vi "运维调试.vi"() -> ()   [LabVIEW 2016]
uses:
  <vilib>/Utility/miscctls.llb/LVPointTypeDef.ctl
  PLC/PLC.lvlib
  <vilib>/Utility/config.llb/NI_LVConfig.lvlib
panel:
  in  "运维调试菜单":T1(xcontrol)
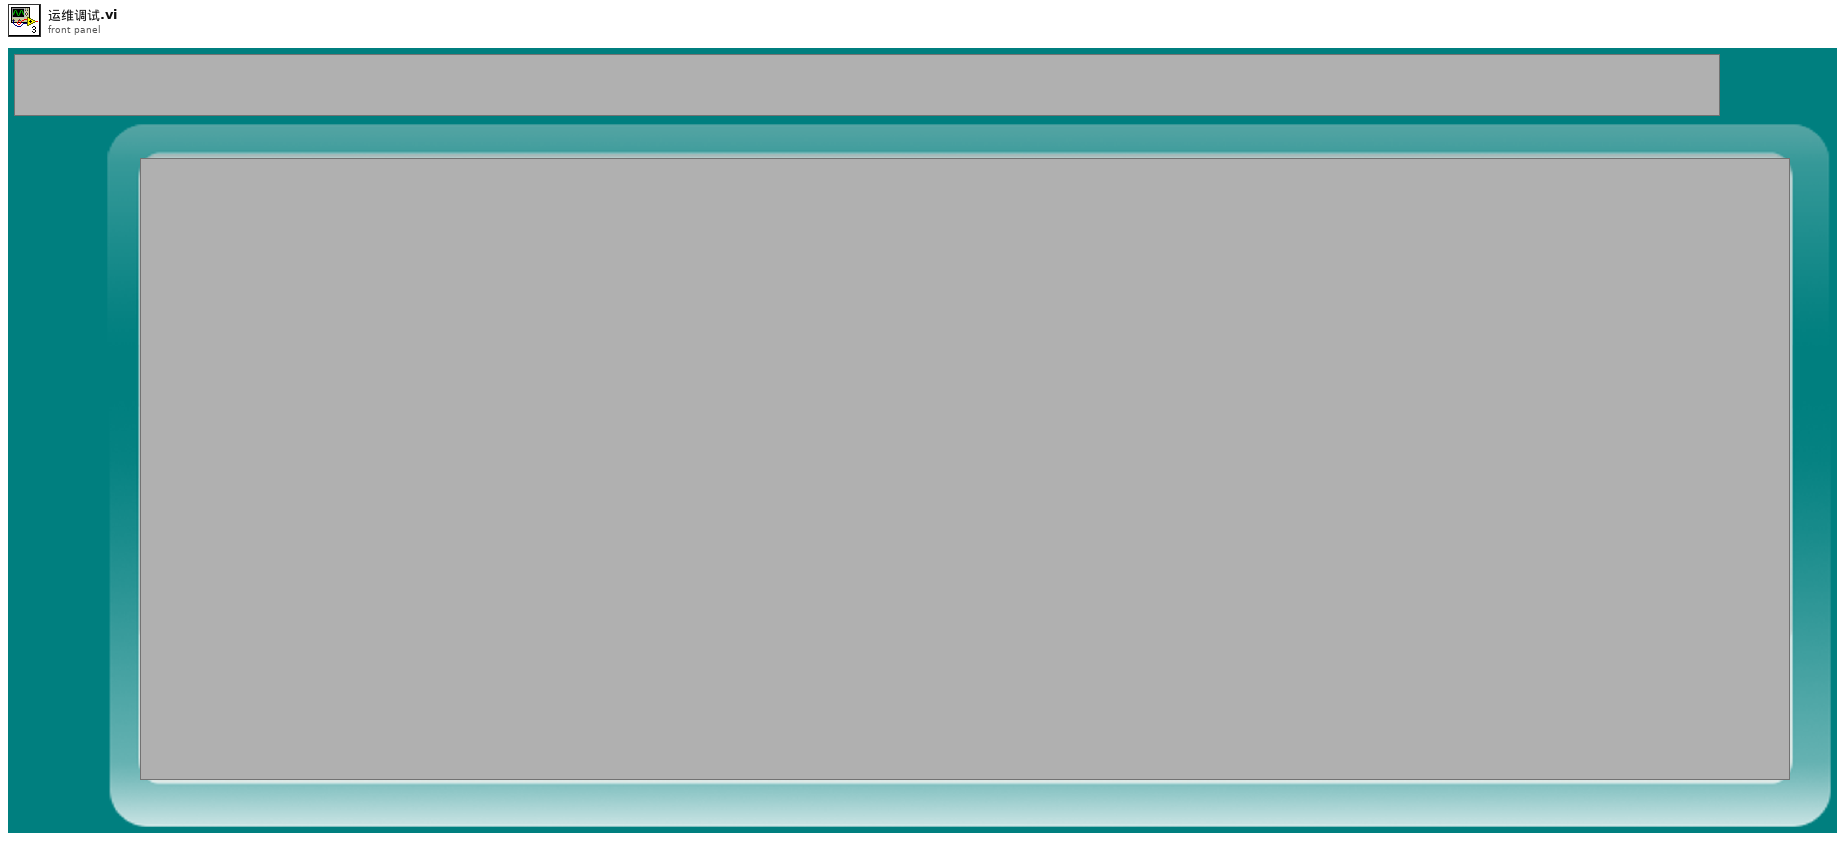
[diagram p1: front panel]
types:
  T1 = enum16{"电源管理", "采配水", "氨氮", "总磷总氮", "多参数", "CODMn", "CODcr", "流量计", "质控单元", "其他"}
  T2 = typedef "NI_LVConfig.lvlib/Config Data RefNum.ctl" = refnum<k1>
  T3 = typedef "LVPointTypeDef.ctl" = cluster{"Horizontal":i16, "Vertical":i16}
  T4 = enum16{"Enabled", "Disabled", "Disabled and Grayed Out"}
  T5 = enum32{"Bad", "Idle", "Run top level", "Running"}
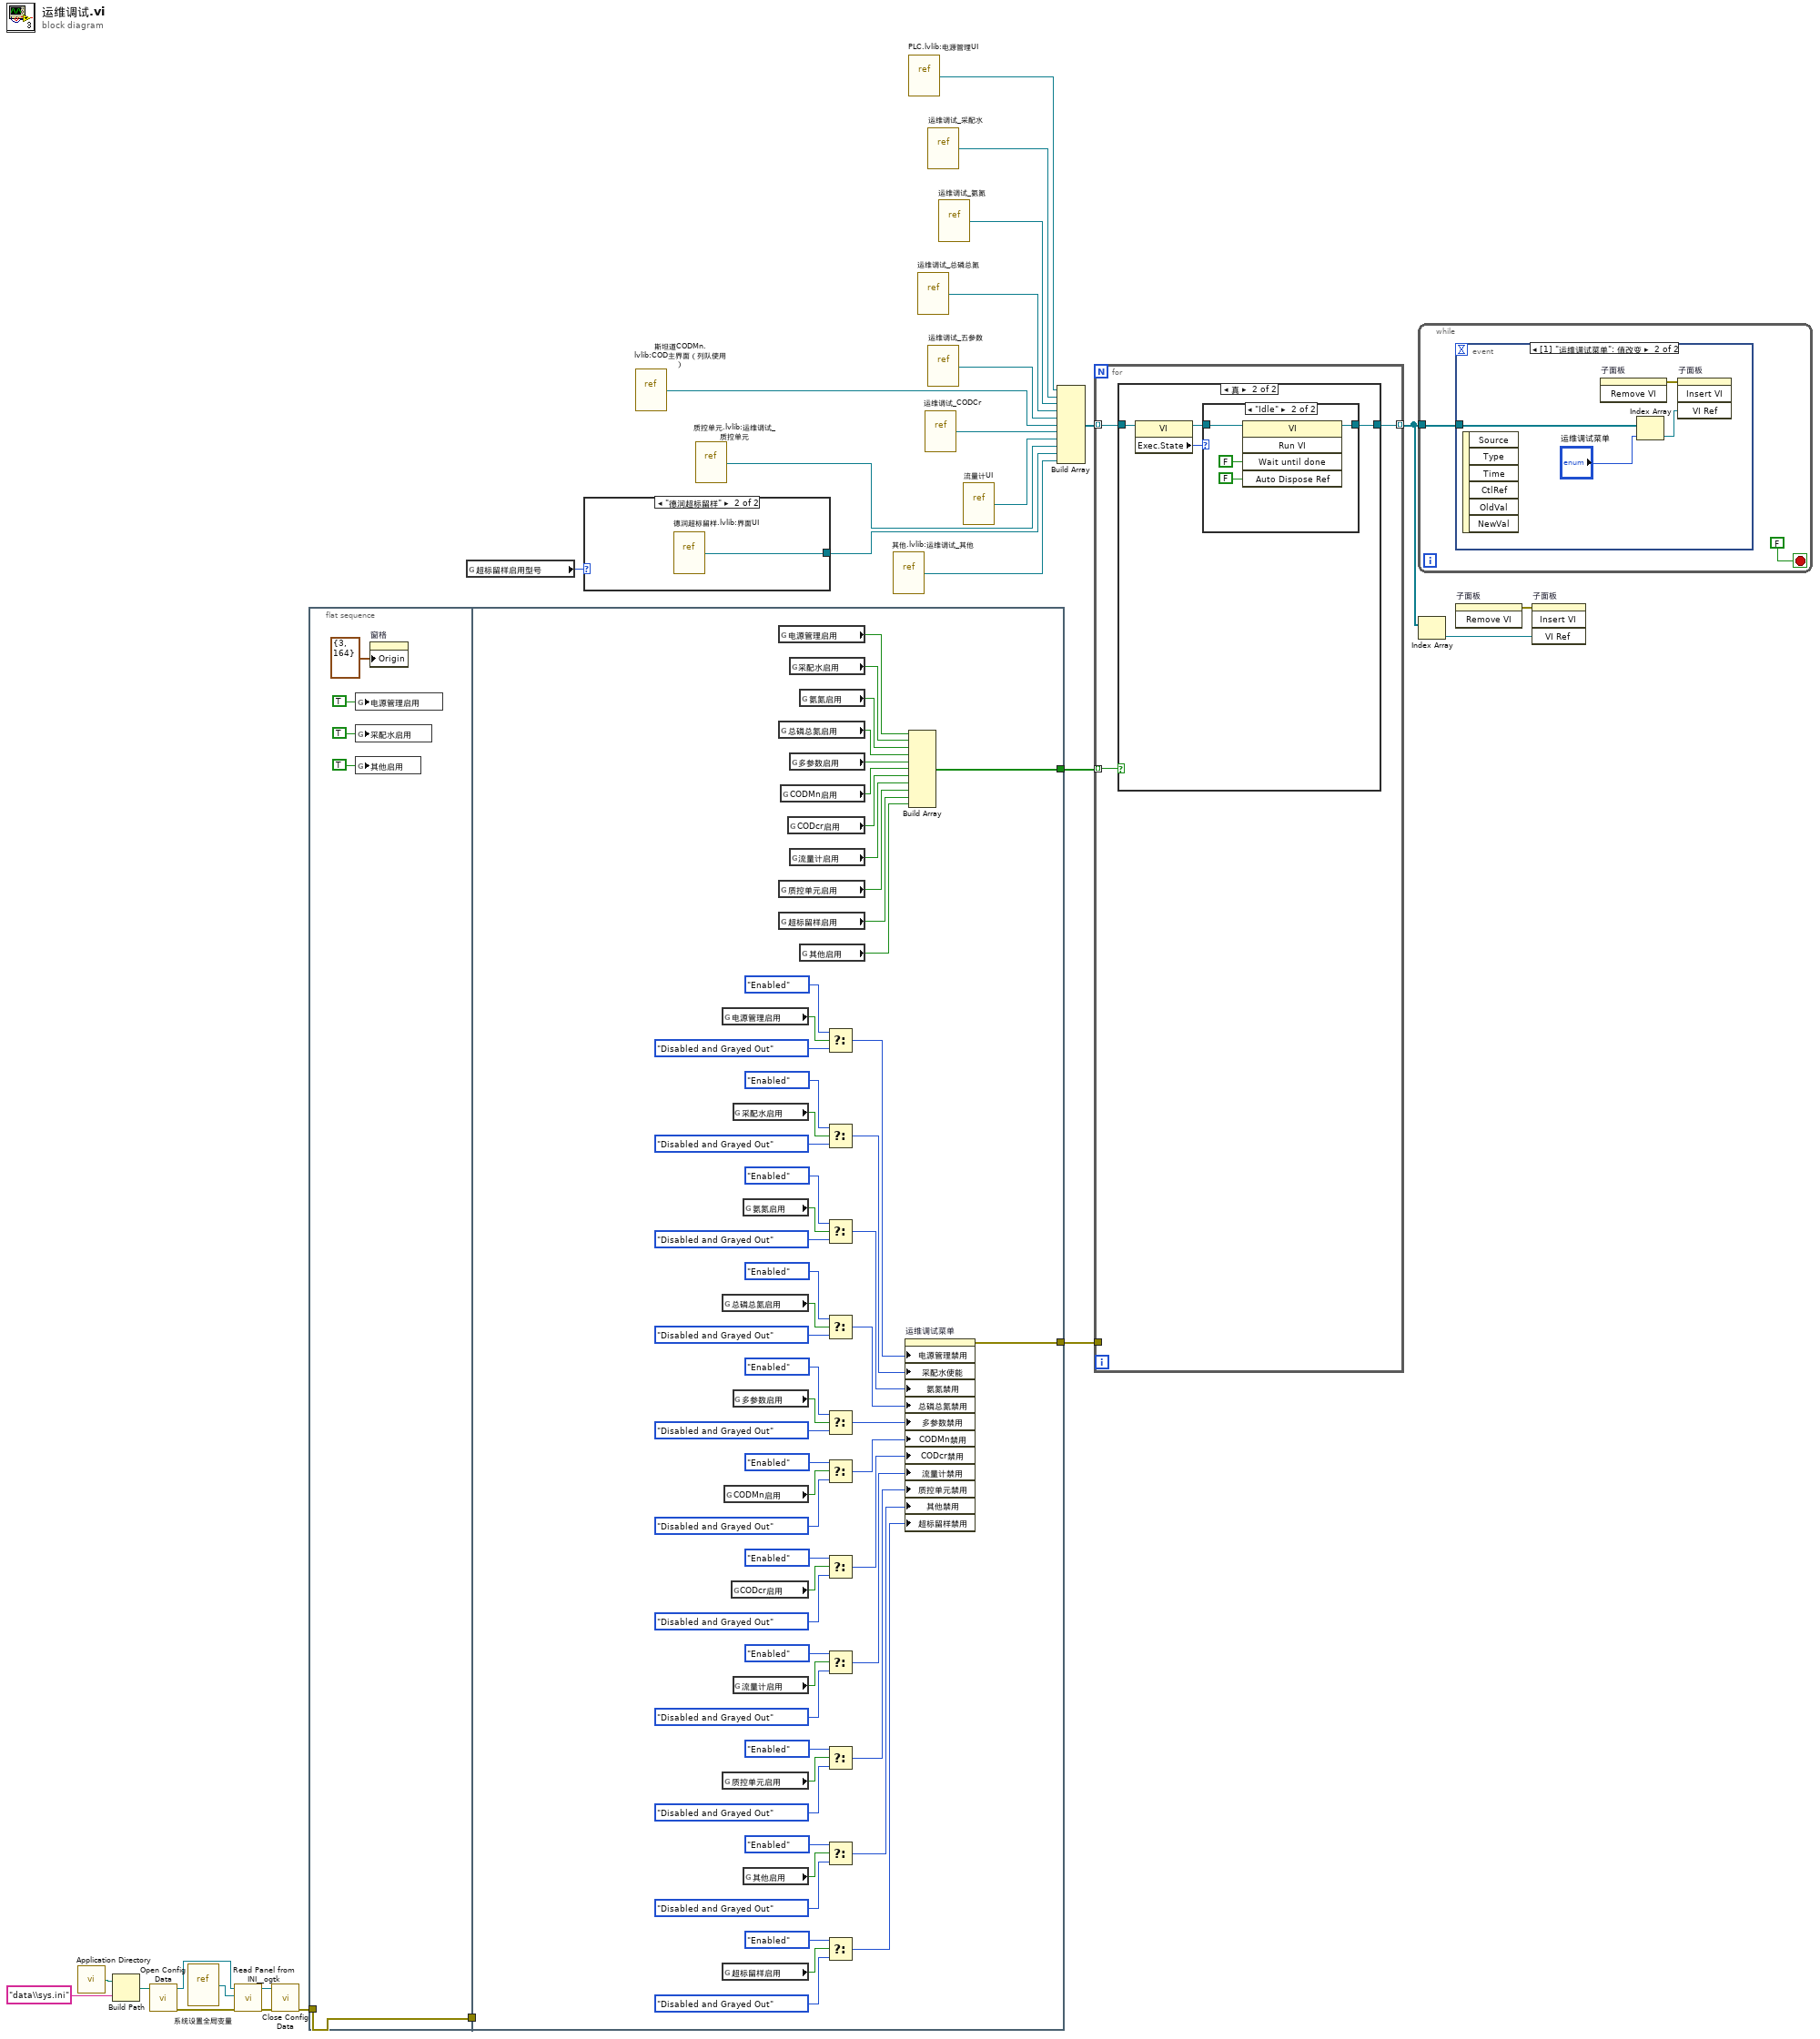
[diagram p0: block diagram]
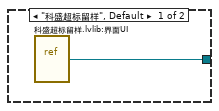
[diagram p2: hidden frame]
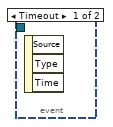
[diagram p5: hidden frame]
diagram:
  n1 = call <vilib>:"Application Directory.vi"() -> ("Application Directory"=w8:path)
  n2 = Build Path(base path=w8, name or relative path="data\\sys.ini" ("名称或相对路径")) -> (appended path=w6:path)
  n3 = call <vilib>:"Open Config Data.vi"("configuration file path"=w6) -> ("error out"=w15:errorcluster, "refnum"=w14:T2)  [unwired: 8 in, 1 out]
  n4 = vi-ref "系统设置全局变量.vi"() -> (w13:refnum<vi>)
  n5 = call <userlib>:"Read Panel from INI__ogtk.vi"("error in (no error)"=w15, "VI ref"=w13, "refnum"=w14) -> ("error out"=w12:errorcluster, "refnum out"=w11:T2)  [unwired: 7 in]
  n6 = call <vilib>:"Close Config Data.vi"("error in (no error)"=w12, "refnum"=w11) -> ("error out"=w10:errorcluster)  [unwired: 8 in, 1 out]
  n7 = flat-sequence {
    tunnel: w10 -> [w33]
    tunnel: [w33] -> w9
    tunnel: [w71] -> w16
    tunnel: w9 -> [_]
    tunnel: [w60] -> w5
    frame #0 {
      n8 = global write "系统设置全局变量.vi" "电源管理启用"(TRUE ("电源管理启用")) -> ()
      n9 = global write "系统设置全局变量.vi" "采配水启用"(TRUE ("采配水启用")) -> ()
      n10 = global write "系统设置全局变量.vi" "其他启用"(TRUE ("其他启用")) -> ()
      n11 = property on="窗格" class="Pane"("Origin"=T3 {"Horizontal"=3, "Vertical"=164} ("原点")) -> ()  [unwired: 2 in, 2 out]
    }
    frame #1 {
      n12 = global read "系统设置全局变量.vi" "电源管理启用"() -> (w90:bool)
      n13 = global read "系统设置全局变量.vi" "总磷总氮启用"() -> (w85:bool)
      n14 = global read "系统设置全局变量.vi" "质控单元启用"() -> (w78:bool)
      n15 = global read "系统设置全局变量.vi" "超标留样启用"() -> (w36:bool)
      n16 = global read "系统设置全局变量.vi" "CODMn启用"() -> (w81:bool)
      n17 = global read "系统设置全局变量.vi" "CODcr启用"() -> (w80:bool)
      n18 = global read "系统设置全局变量.vi" "采配水启用"() -> (w87:bool)
      n19 = global read "系统设置全局变量.vi" "多参数启用"() -> (w83:bool)
      n20 = global read "系统设置全局变量.vi" "流量计启用"() -> (w79:bool)
      n21 = global read "系统设置全局变量.vi" "氨氮启用"() -> (w39:bool)
      n22 = global read "系统设置全局变量.vi" "其他启用"() -> (w77:bool)
      n23 = global read "系统设置全局变量.vi" "电源管理启用"() -> (w61:bool)
      n24 = global read "系统设置全局变量.vi" "总磷总氮启用"() -> (w64:bool)
      n25 = global read "系统设置全局变量.vi" "质控单元启用"() -> (w69:bool)
      n26 = global read "系统设置全局变量.vi" "超标留样启用"() -> (w70:bool)
      n27 = global read "系统设置全局变量.vi" "CODMn启用"() -> (w66:bool)
      n28 = global read "系统设置全局变量.vi" "CODcr启用"() -> (w67:bool)
      n29 = global read "系统设置全局变量.vi" "采配水启用"() -> (w62:bool)
      n30 = global read "系统设置全局变量.vi" "多参数启用"() -> (w65:bool)
      n31 = global read "系统设置全局变量.vi" "流量计启用"() -> (w68:bool)
      n32 = global read "系统设置全局变量.vi" "氨氮启用"() -> (w63:bool)
      n33 = global read "系统设置全局变量.vi" "其他启用"() -> (w34:bool)
      n34 = Select(t=T4."Enabled" ("电源管理禁用"), s=w90, f=T4."Disabled and Grayed Out" ("电源管理禁用")) -> (s? t:f=w89:T4)
      n35 = Select(t=T4."Enabled" ("电源管理禁用"), s=w87, f=T4."Disabled and Grayed Out" ("电源管理禁用")) -> (s? t:f=w88:T4)
      n36 = Select(t=T4."Enabled" ("电源管理禁用"), s=w39, f=T4."Disabled and Grayed Out" ("电源管理禁用")) -> (s? t:f=w86:T4)
      n37 = Select(t=T4."Enabled" ("电源管理禁用"), s=w85, f=T4."Disabled and Grayed Out" ("电源管理禁用")) -> (s? t:f=w84:T4)
      n38 = Select(t=T4."Enabled" ("电源管理禁用"), s=w83, f=T4."Disabled and Grayed Out" ("电源管理禁用")) -> (s? t:f=w82:T4)
      n39 = Select(t=T4."Enabled" ("电源管理禁用"), s=w81, f=T4."Disabled and Grayed Out" ("电源管理禁用")) -> (s? t:f=w76:T4)
      n40 = Select(t=T4."Enabled" ("电源管理禁用"), s=w80, f=T4."Disabled and Grayed Out" ("电源管理禁用")) -> (s? t:f=w75:T4)
      n41 = Select(t=T4."Enabled" ("电源管理禁用"), s=w79, f=T4."Disabled and Grayed Out" ("电源管理禁用")) -> (s? t:f=w74:T4)
      n42 = Select(t=T4."Enabled" ("电源管理禁用"), s=w78, f=T4."Disabled and Grayed Out" ("电源管理禁用")) -> (s? t:f=w73:T4)
      n43 = Select(t=T4."Enabled" ("电源管理禁用"), s=w77, f=T4."Disabled and Grayed Out" ("电源管理禁用")) -> (s? t:f=w72:T4)
      n44 = Select(t=T4."Enabled" ("电源管理禁用"), s=w36, f=T4."Disabled and Grayed Out" ("电源管理禁用")) -> (s? t:f=w35:T4)
      n45 = property on="运维调试菜单" class="运维调试菜单 (严格)"("电源管理禁用"=w89, "采配水使能"=w88, "氨氮禁用"=w86, "总磷总氮禁用"=w84, "多参数禁用"=w82, "CODMn禁用"=w76, "CODcr禁用"=w75, "流量计禁用"=w74, "质控单元禁用"=w73, "其他禁用"=w72, "超标留样禁用"=w35) -> (error out=w71:errorcluster)  [unwired: 2 in, 1 out]
      n46 = Build Array(w61, w62, w63, w64, w65, w66, w67, w68, w69, w70, w34) -> (w60:bool[])
    }
  }
  n47 = global read "系统设置全局变量.vi" "超标留样启用型号"() -> (w2:enum16{"科盛超标留样", "德润超标留样"})
  n48 = case shown="\"德润超标留样\"" w2 {
    tunnel: [w91 w92] -> w1
    frame "科盛超标留样", Default {
      n49 = vi-ref "科盛超标留样.lvlib:界面UI.vi"() -> (w91:refnum<vi>)
    }
    frame "德润超标留样" {
      n50 = vi-ref "德润超标留样.lvlib:界面UI.vi"() -> (w92:refnum<vi>)
    }
  }
  n51 = vi-ref "斯坦道CODMn.lvlib:COD主界面（列队使用）.vi"() -> (w21:refnum<vi>)
  n52 = vi-ref "质控单元.lvlib:运维调试_质控单元.vi"() -> (w19:refnum<vi>)
  n53 = vi-ref "其他.lvlib:运维调试_其他.vi"() -> (w3:refnum<vi>)
  n54 = vi-ref "PLC.lvlib:电源管理UI.vi"() -> (w18:refnum<vi>)
  n55 = vi-ref "运维调试_总磷总氮.vi"() -> (w23:refnum<vi>)
  n56 = vi-ref "运维调试_CODCr.vi"() -> (w20:refnum<vi>)
  n57 = vi-ref "运维调试_采配水.vi"() -> (w24:refnum<vi>)
  n58 = vi-ref "运维调试_五参数.vi"() -> (w22:refnum<vi>)
  n59 = vi-ref "运维调试_氨氮.vi"() -> (w4:refnum<vi>)
  n60 = vi-ref "流量计UI.vi"() -> (w17:refnum<vi>)
  n61 = Build Array(w18, w24, w4, w23, w22, w21, w20, w17, w19, w1, w3) -> (w25:refnum<vi>[])
  n62 = for {
    tunnel: w25 -> [w95] mode=indexing
    tunnel: [w94] -> w27 mode=indexing
    tunnel: w5 -> [w93] mode=indexing
    tunnel: w16 -> [_]
    n63 = case shown="真" w93 {
      tunnel: w95 -> [w96 w100]
      tunnel: [w96 w97] -> w94
      frame False {
      }
      frame True {
        n64 = property class="VI"(reference=w100) -> (reference out=w98:refnum<vi>, "Exec.State"=w99:T5)  [unwired: 1 in, 1 out]
        n65 = case shown="\"Idle\"" w99 {
          tunnel: w98 -> [w101 w103]
          tunnel: [w101 w102] -> w97
          frame "Bad", Default {
          }
          frame "Idle" {
            n66 = invoke class="VI" method="Run VI"(reference=w103, "Wait until done"=FALSE ("结束前等待"), "Auto Dispose Ref"=FALSE ("自动销毁引用")) -> (reference out=w102:refnum<vi>)  [unwired: 2 in, 4 out]
          }
        }
      }
    }
  }
  n67 = while {
    tunnel: w27 -> [w106]
    stop <- FALSE stop-if-true
    n68 = event shown="[1] \"运维调试菜单\": 值改变" {
      selector: _ -> [_ _]
      dyn-events: _ -> [_ _]
      timeout: _ -> [_ _]
      tunnel: w106 -> [_ w110]
      event Timeout {
        n69 = event-data() -> ()  [unwired: 1 in, 3 out]
      }
      event "运维调试菜单": Value Change {
        n70 = event-data() -> ()  [unwired: 1 in, 6 out]
        n71 = invoke on="子面板" class="SubPnl" method="Remove VI"() -> (error out=w111:errorcluster)  [unwired: 3 in, 2 out]
        n72 = Index Array(array=w110, index="运维调试菜单") -> (element=w109:refnum<vi>)
        n73 = invoke on="子面板" class="SubPnl" method="Insert VI"(error in=w111, "VI Ref"=w109) -> ()  [unwired: 2 in, 4 out]
      }
    }
  }
  n74 = Index Array(array=w27) -> (element=w26:refnum<vi>)  [unwired: 1 in]
  n75 = invoke on="子面板" class="SubPnl" method="Remove VI"() -> (error out=w28:errorcluster)  [unwired: 3 in, 2 out]
  n76 = invoke on="子面板" class="SubPnl" method="Insert VI"(error in=w28, "VI Ref"=w26) -> ()  [unwired: 2 in, 4 out]
